vi "Fix Title Strings.vi"(1 "Title In":string[](array[string])) -> (0 "Title Out":string[](array[string]))   [LabVIEW 2020]
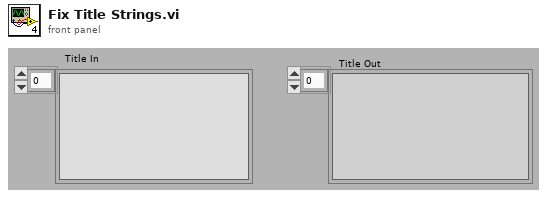
[diagram p1: front panel]
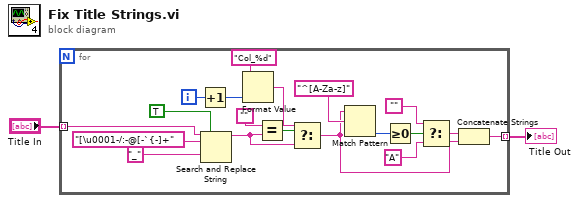
[diagram p0: block diagram]
diagram:
  n1 = for {
    tunnel: "Title In" -> [w12] mode=indexing
    tunnel: [w4] -> w2 mode=indexing
    i -> [w3]
    n2 = Increment(x=w3) -> (x+1=w7:i32)
    n3 = Search and Replace String(replace all?=TRUE ("replace all? (F)"), input string=w12, search string="[\u0001-/:-@[-`{-]+", replace string="_" ("replace string (\"\")")) -> (result string=w6:string)  [unwired: 4 in, 3 out]
    n4 = Format Value(format string="Col_%d", value (0)=w7) -> (output string=w9:string)  [unwired: 1 in]
    n5 = Equal?(x="", y=w6) -> (x = y?=w10:bool)
    n6 = Select(t=w9, s=w10, f=w6) -> (s? t:f=w5:string)
    n7 = Match Pattern(string=w5, regular expression="^[A-Za-z]") -> (offset past match=w17:i32)  [unwired: 1 in, 3 out]
    n8 = Greater Or Equal To 0?(x=w17) -> (x >= 0?=w18:bool)
    n9 = Select(t="", s=w18, f="A" ("regular expression")) -> (s? t:f=w21:string)
    n10 = Concatenate Strings(w21, w5) -> (w4:string)
  }
  "Title Out" <- w2
